vi "Test_uart.vi"() -> ()   [LabVIEW 2025]
uses:
  <vilib>/Instr/_visa.llb/VISA Configure Serial Port (Instr).vi
panel:
  in  "Enviar Stats":bool
  in  "Stats":T1={"Engranes"=90.0, "Pulsos"=22, "MAX_RPM"=110}
  in  "Enviar":bool
  in  "Stop Button":bool
  out "Waveform Chart":T2(graph)
  in  "Tab Control":T3(tab)
  out "PWM_num":dbl
  in  "PWM":dbl(slide) scale=0.0..999.0
  in  "Cuad":T4 {"Tiempo en Min" step=10; "Tiempo en Max" step=10}
  in  "Triag":T5
  in  "Diente":T5
  in  "Ramp":T5
  # "ms"
  # "ms"
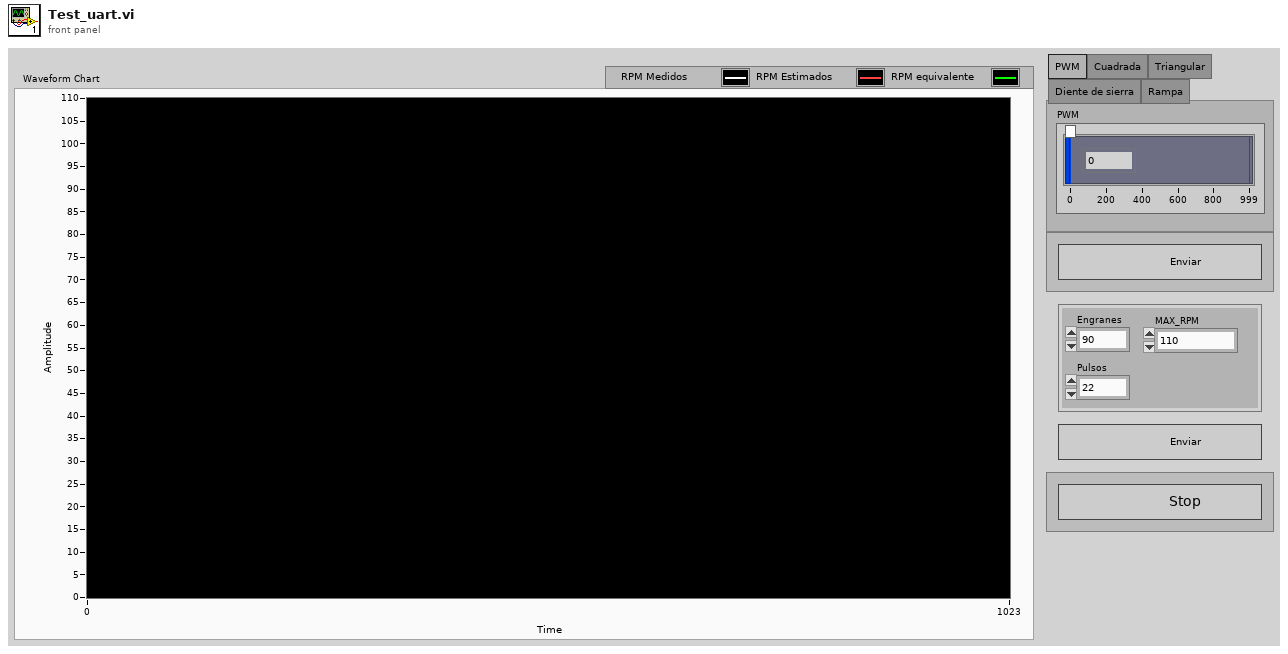
[diagram p1: front panel]
types:
  T1 = cluster{"Engranes":sgl, "Pulsos":u16, "MAX_RPM":u16}
  T2 = cluster{"Número":sgl, "Número":sgl, "Número":sgl}
  T3 = enum32{"PWM", "Cuadrada", "Triangular", "Diente de sierra", "Rampa"}
  T4 = cluster{"Maximo":u16, "Minimo":u16, "Tiempo en Max":u16, "Tiempo en Min":u16}
  T5 = cluster{"Maximo":u16, "Minimo":u16, "Aumento Y":u16, "Aumento X":u16}
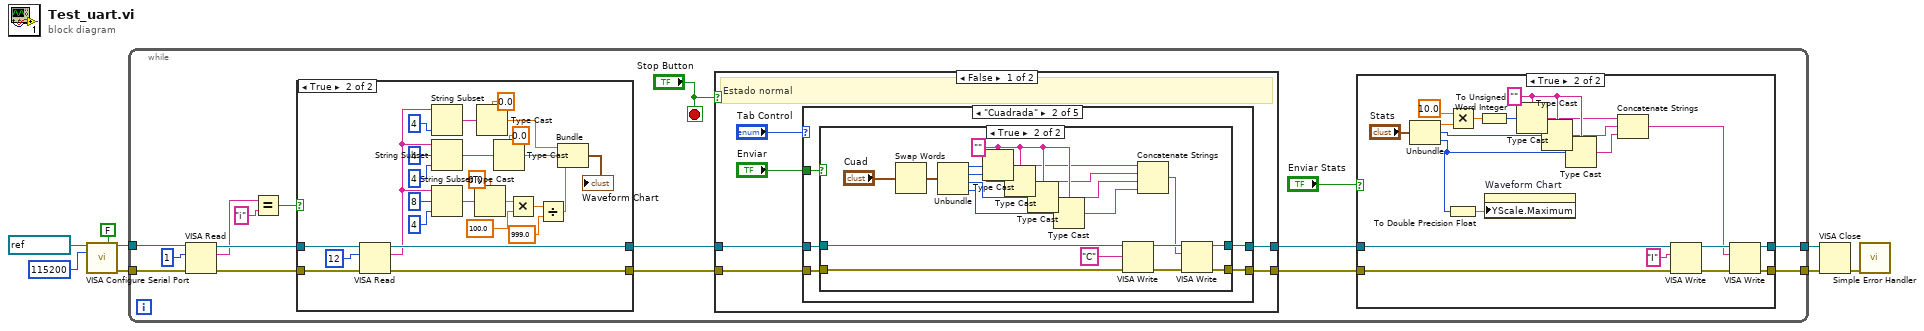
[diagram p0: block diagram]
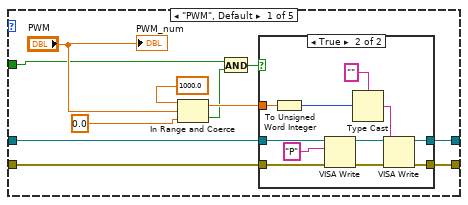
[diagram p3: hidden frame]
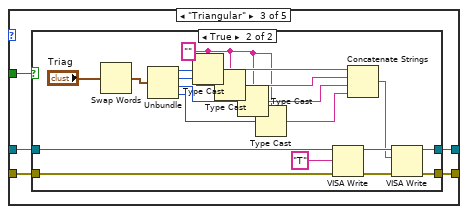
[diagram p6: hidden frame]
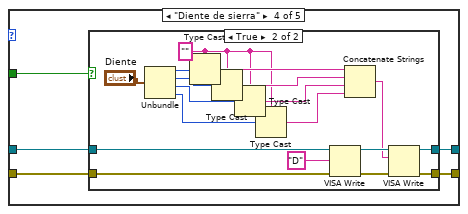
[diagram p8: hidden frame]
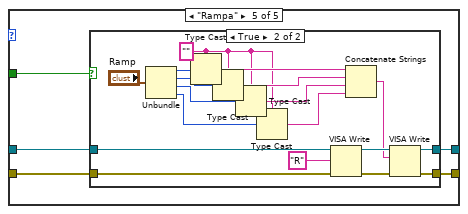
[diagram p10: hidden frame]
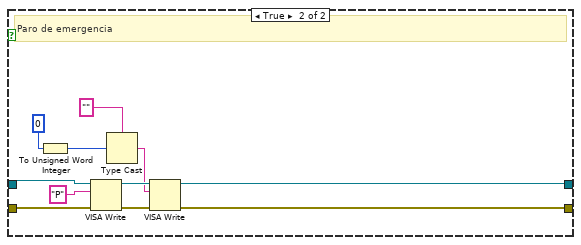
[diagram p12: hidden frame]
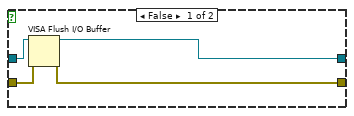
[diagram p13: hidden frame]
diagram:
  n1 = call-poly "VISA Configure Serial Port"("VISA resource name"=refnum<visa-resource-name> "COM4", "Enable Termination\nChar (T)"=FALSE ("Enable Termination\nChar (T)"), "baud rate (9600)"=u32 115200) -> ("VISA resource name out"=w3:refnum<visa-resource-name>, "error out"=w2:errorcluster)  [unwired: 11 in]
  n2 = while {
    tunnel: w3 -> [w23]
    tunnel: w2 -> [w22]
    tunnel: [w11] -> w8
    tunnel: [w10] -> w7
    stop <- "Stop Button" stop-if-true
    n3 = VISA Read(VISA resource name=w23, byte count=u32 1, error in (no error)=w22) -> (VISA resource name out=w21:refnum<visa-resource-name>, read buffer=w19:string, error out=w20:errorcluster)  [unwired: 1 out]
    n4 = Equal?(x=w19, y="i") -> (x = y?=w17:bool)
    n5 = case shown="True" w17 {
      tunnel: [w193 w218] -> w16
      tunnel: [w192 w217] -> w15
      tunnel: w21 -> [w191 w214]
      tunnel: w20 -> [w190 w213]
      frame False {
        n6 = VISA Flush I/O Buffer(VISA resource name=w191, error in (no error)=w190) -> (VISA resource name out=w193:refnum<visa-resource-name>, error out=w192:errorcluster)  [unwired: 1 in]
      }
      frame True {
        n7 = VISA Read(VISA resource name=w214, byte count=u32 12, error in (no error)=w213) -> (VISA resource name out=w218:refnum<visa-resource-name>, read buffer=w202:string, error out=w217:errorcluster)  [unwired: 1 out]
        n8 = String Subset(string=w202, length (rest)=4 ("length (rest)")) -> (substring=w211:string)  [unwired: 1 in]
        n9 = String Subset(string=w202, offset (0)=4, length (rest)=4 ("length (rest)")) -> (substring=w205:string)
        n10 = String Subset(string=w202, offset (0)=8, length (rest)=4 ("length (rest)")) -> (substring=w201:string)
        n11 = Type Cast(type=sgl 0.0 ("Número"), x=w201) -> (*(type *) &x=w199:sgl)
        n12 = Type Cast(type=sgl 0.0 ("Número"), x=w211) -> (*(type *) &x=w208:sgl)
        n13 = Type Cast(type=sgl 0.0 ("Número"), x=w205) -> (*(type *) &x=w206:sgl)
        n14 = Multiply(x=w199, y=sgl 100.0) -> (x*y=w197:sgl)
        n15 = Divide(x=w197, y=sgl 999.0) -> (x/y=w195:sgl)
        n16 = Bundle("Número"=w208, "Número"=w206, w195) -> (→"Waveform Chart":cluster{"Número":sgl, "Número":sgl, sgl})  [unwired: 1 in]
      }
    }
    n17 = case shown="False" "Stop Button" {
      tunnel: w16 -> [w51 w183]
      tunnel: w15 -> [w50 w182]
      tunnel: [w49 w181] -> w13
      tunnel: [w48 w180] -> w12
      frame False {
        # "Estado normal"
        n18 = case shown="\"Cuadrada\"" "Tab Control" {
          tunnel: w51 -> [w59 w81 w107 w133 w158]
          tunnel: w50 -> [w58 w80 w106 w132 w157]
          tunnel: [w57 w79 w105 w131 w156] -> w49
          tunnel: [w56 w78 w104 w130 w155] -> w48
          tunnel: "Enviar" -> [w53 w77 w103 w129 w154]
          frame "PWM", Default {
            n19 = In Range and Coerce(upper limit=1000.0, x="PWM", lower limit=0.0) -> (coerced(x)=w63:dbl, In Range?=w62:bool)
            n20 = And(x=w53, y=w62) -> (x .and. y?=w55:bool)
            n21 = case shown="True" w55 {
              tunnel: w59 -> [w65 w76]
              tunnel: w58 -> [w64 w75]
              tunnel: w63 -> [_ w67]
              tunnel: [w65 w71] -> w57
              tunnel: [w64 w70] -> w56
              frame False {
              }
              frame True {
                n22 = To Unsigned Word Integer(number=w67) -> (unsigned 16bit integer=w66:u16)
                n23 = VISA Write(VISA resource name=w76, write buffer="P", error in (no error)=w75) -> (VISA resource name out=w72:refnum<visa-resource-name>, error out=w73:errorcluster)  [unwired: 1 out]
                n24 = Type Cast(type="", x=w66) -> (*(type *) &x=w69:string)
                n25 = VISA Write(VISA resource name=w72, write buffer=w69, error in (no error)=w73) -> (VISA resource name out=w71:refnum<visa-resource-name>, error out=w70:errorcluster)  [unwired: 1 out]
              }
            }
            "PWM_num" <- "PWM"
          }
          frame "Cuadrada" {
            n26 = case shown="True" w77 {
              tunnel: w81 -> [w83 w102]
              tunnel: w80 -> [w82 w101]
              tunnel: [w83 w98] -> w79
              tunnel: [w82 w97] -> w78
              frame False {
              }
              frame True {
                w94 = ""
                n27 = Swap Words(1:"Cuad") -> (0:w84:T4)
                n28 = Unbundle(w84) -> ("Maximo"=w96:u16, "Minimo"=w93:u16, "Tiempo en Max"=w92:u16, "Tiempo en Min"=w91:u16)
                n29 = Type Cast(type=w94, x=w96) -> (*(type *) &x=w90:string)
                n30 = Type Cast(type=w94, x=w93) -> (*(type *) &x=w88:string)
                n31 = Type Cast(type=w94, x=w92) -> (*(type *) &x=w87:string)
                n32 = Type Cast(type=w94, x=w91) -> (*(type *) &x=w86:string)
                n33 = VISA Write(VISA resource name=w102, write buffer="C", error in (no error)=w101) -> (VISA resource name out=w99:refnum<visa-resource-name>, error out=w100:errorcluster)  [unwired: 1 out]
                n34 = Concatenate Strings(w90, w88, w87, w86) -> (w89:string)
                n35 = VISA Write(VISA resource name=w99, write buffer=w89, error in (no error)=w100) -> (VISA resource name out=w98:refnum<visa-resource-name>, error out=w97:errorcluster)  [unwired: 1 out]
              }
            }
          }
          frame "Triangular" {
            n36 = case shown="True" w103 {
              tunnel: w107 -> [w109 w128]
              tunnel: w106 -> [w108 w127]
              tunnel: [w109 w124] -> w105
              tunnel: [w108 w123] -> w104
              frame False {
              }
              frame True {
                w111 = ""
                n37 = Swap Words(1:"Triag") -> (0:w113:T5)
                n38 = Unbundle(w113) -> ("Maximo"=w122:u16, "Minimo"=w120:u16, "Aumento Y"=w119:u16, "Aumento X"=w110:u16)
                n39 = Type Cast(type=w111, x=w122) -> (*(type *) &x=w118:string)
                n40 = Type Cast(type=w111, x=w120) -> (*(type *) &x=w115:string)
                n41 = Type Cast(type=w111, x=w119) -> (*(type *) &x=w116:string)
                n42 = Type Cast(type=w111, x=w110) -> (*(type *) &x=w112:string)
                n43 = VISA Write(VISA resource name=w128, write buffer="T", error in (no error)=w127) -> (VISA resource name out=w125:refnum<visa-resource-name>, error out=w126:errorcluster)  [unwired: 1 out]
                n44 = Concatenate Strings(w118, w115, w116, w112) -> (w117:string)
                n45 = VISA Write(VISA resource name=w125, write buffer=w117, error in (no error)=w126) -> (VISA resource name out=w124:refnum<visa-resource-name>, error out=w123:errorcluster)  [unwired: 1 out]
              }
            }
          }
          frame "Diente de sierra" {
            n46 = case shown="True" w129 {
              tunnel: w133 -> [w135 w153]
              tunnel: w132 -> [w134 w152]
              tunnel: [w135 w149] -> w131
              tunnel: [w134 w148] -> w130
              frame False {
              }
              frame True {
                w137 = ""
                n47 = Unbundle("Diente") -> ("Maximo"=w147:u16, "Minimo"=w145:u16, "Aumento Y"=w144:u16, "Aumento X"=w136:u16)
                n48 = Type Cast(type=w137, x=w147) -> (*(type *) &x=w143:string)
                n49 = Type Cast(type=w137, x=w145) -> (*(type *) &x=w141:string)
                n50 = Type Cast(type=w137, x=w144) -> (*(type *) &x=w140:string)
                n51 = Type Cast(type=w137, x=w136) -> (*(type *) &x=w138:string)
                n52 = VISA Write(VISA resource name=w153, write buffer="D", error in (no error)=w152) -> (VISA resource name out=w150:refnum<visa-resource-name>, error out=w151:errorcluster)  [unwired: 1 out]
                n53 = Concatenate Strings(w143, w141, w140, w138) -> (w142:string)
                n54 = VISA Write(VISA resource name=w150, write buffer=w142, error in (no error)=w151) -> (VISA resource name out=w149:refnum<visa-resource-name>, error out=w148:errorcluster)  [unwired: 1 out]
              }
            }
          }
          frame "Rampa" {
            n55 = case shown="True" w154 {
              tunnel: w158 -> [w160 w178]
              tunnel: w157 -> [w159 w177]
              tunnel: [w160 w174] -> w156
              tunnel: [w159 w173] -> w155
              frame False {
              }
              frame True {
                w161 = ""
                n56 = Unbundle("Ramp") -> ("Maximo"=w172:u16, "Minimo"=w170:u16, "Aumento Y"=w169:u16, "Aumento X"=w162:u16)
                n57 = Type Cast(type=w161, x=w172) -> (*(type *) &x=w168:string)
                n58 = Type Cast(type=w161, x=w170) -> (*(type *) &x=w166:string)
                n59 = Type Cast(type=w161, x=w169) -> (*(type *) &x=w165:string)
                n60 = Type Cast(type=w161, x=w162) -> (*(type *) &x=w163:string)
                n61 = VISA Write(VISA resource name=w178, write buffer="R", error in (no error)=w177) -> (VISA resource name out=w175:refnum<visa-resource-name>, error out=w176:errorcluster)  [unwired: 1 out]
                n62 = Concatenate Strings(w168, w166, w165, w163) -> (w167:string)
                n63 = VISA Write(VISA resource name=w175, write buffer=w167, error in (no error)=w176) -> (VISA resource name out=w174:refnum<visa-resource-name>, error out=w173:errorcluster)  [unwired: 1 out]
              }
            }
          }
        }
      }
      frame True {
        # "Paro de emergencia"
        n64 = To Unsigned Word Integer(number=u16 0) -> (unsigned 16bit integer=w186:u16)
        n65 = VISA Write(VISA resource name=w183, write buffer="P", error in (no error)=w182) -> (VISA resource name out=w187:refnum<visa-resource-name>, error out=w188:errorcluster)  [unwired: 1 out]
        n66 = Type Cast(type="", x=w186) -> (*(type *) &x=w185:string)
        n67 = VISA Write(VISA resource name=w187, write buffer=w185, error in (no error)=w188) -> (VISA resource name out=w181:refnum<visa-resource-name>, error out=w180:errorcluster)  [unwired: 1 out]
      }
    }
    n68 = case shown="True" "Enviar Stats" {
      tunnel: w13 -> [w26 w31]
      tunnel: w12 -> [w25 w30]
      tunnel: [w26 w35] -> w11
      tunnel: [w25 w36] -> w10
      frame False {
      }
      frame True {
        w40 = ""
        n69 = Unbundle("Stats") -> ("Engranes"=w45:sgl, "Pulsos"=w41:u16, "MAX_RPM"=w27:u16)
        n70 = Multiply(x=sgl 10.0, y=w45) -> (x*y=w43:sgl)
        n71 = To Double Precision Float(number=w27) -> (double precision float=w28:dbl)
        n72 = To Unsigned Word Integer(number=w43) -> (unsigned 16bit integer=w42:u16)
        n73 = property on="Waveform Chart" class="WFChart (strict)"("YScale.Maximum"=w28) -> ()  [unwired: 2 in, 2 out]
        n74 = Type Cast(type=w40, x=w42) -> (*(type *) &x=w39:string)
        n75 = Type Cast(type=w40, x=w41) -> (*(type *) &x=w38:string)
        n76 = Type Cast(type=w40, x=w27) -> (*(type *) &x=w37:string)
        n77 = Concatenate Strings(w39, w38, w37) -> (w32:string)
        n78 = VISA Write(VISA resource name=w31, write buffer="I", error in (no error)=w30) -> (VISA resource name out=w34:refnum<visa-resource-name>, error out=w33:errorcluster)  [unwired: 1 out]
        n79 = VISA Write(VISA resource name=w34, write buffer=w32, error in (no error)=w33) -> (VISA resource name out=w35:refnum<visa-resource-name>, error out=w36:errorcluster)  [unwired: 1 out]
      }
    }
  }
  n80 = VISA Close(VISA resource name=w8, error in (no error)=w7) -> (error out=w1:errorcluster)
  n81 = call <vilib>:"Simple Error Handler.vi"("error in (no error)"=w1) -> ()  [unwired: 4 in, 5 out]
